vi "Parse Version String from Git.vi"(8 "error in":errorcluster, 11 "Version String":string) -> (0 "error out":errorcluster, 1 "Commit Hash":string, 2 "Version":cluster{i32, i32, i32, i32})   [LabVIEW 2019]
uses:
  <vilib>/Utility/error.llb/Error Cluster From Error Code.vi
  <vilib>/regexp/Match Regular Expression.xnode
  <vilib>/ErrorRing/Error Ring.xnode
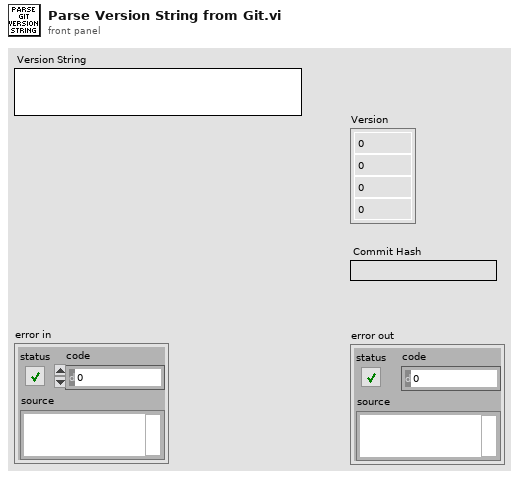
[diagram p1: front panel]
types:
  T1 = cluster{"[0]":i32, "[1]":i32, "[2]":i32, "[3]":i32}
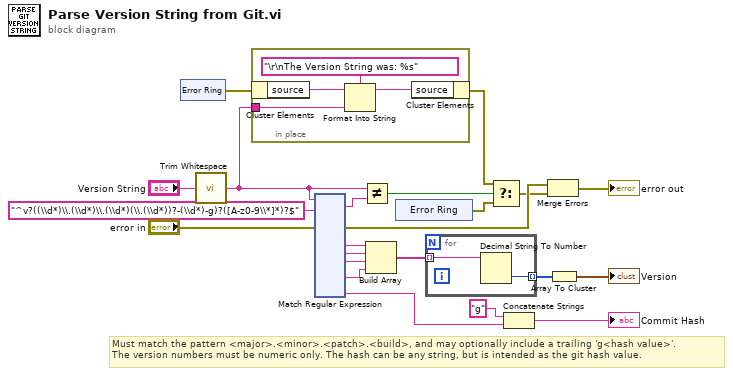
[diagram p0: block diagram]
diagram:
  # "Must match the pattern <major>.<minor>.<patch>.<build>, and may optionally include a trailing 'g<hash value>'.\nThe version numbers must be numeric only. The hash can be any string, but is intended as the git hash value."
  n1 = xnode "Error Ring"() -> ("error out"=w8:errorcluster)
  n2 = call <vilib>:"Trim Whitespace.vi"("string"="Version String") -> ("trimmed string"=w2:string)  [unwired: 1 in]
  n3 = in-place {
    in-place-border: w2 -> [w24]
    n4 = in-place-cluster #1(w8) -> ("source"=w26:string)
    n5 = Format Into String(format string="\r\nThe Version String was: %s", initial string=w26, w24) -> (resulting string=w25:string)  [unwired: 1 in, 1 out]
    n6 = in-place-cluster #1("source"=w25) -> (w7:errorcluster)
  }
  n7 = xnode "Match Regular Expression"("input string"=w2, "regular expression"="^v?((\\d*)\\.(\\d*)\\.(\\d*)(\\.(\\d*))?-(\\d*)-g)?([A-z0-9\\*]*)?$", "error in"="error in") -> ("whole match"=w18:string, "error out"=w15:errorcluster, "submatch 2"=w12:string, "submatch 3"=w11:string, "submatch 4"=w10:string, "submatch 6"=w5:string, "submatch 8"=w6:string)  [unwired: 3 in, 6 out]
  n8 = Not Equal?(x=w2, y=w18) -> (x != y?=w16:bool)
  n9 = Build Array(w12, w11, w10, w5) -> (w21:string[])
  n10 = xnode "Error Ring"() -> ("error out"=w13:errorcluster)
  n11 = for {
    tunnel: w21 -> [w28] mode=indexing
    tunnel: [w27] -> w20 mode=indexing
    n12 = Decimal String To Number(string=w28) -> (number=w27:i32)  [unwired: 2 in, 1 out]
  }
  n13 = Select(t=w7, s=w16, f=w13) -> (s? t:f=w9:errorcluster)
  n14 = Concatenate Strings("g" ("string"), w6) -> (→"Commit Hash":string)
  n15 = Merge Errors(w15, w9) -> (→"error out":errorcluster)
  n16 = Array To Cluster(array=w20) -> (cluster=→"Version":T1)
